vi "Random_Number.vi"() -> ()   [LabVIEW 2017]
panel:
  in  "stop":bool
  out "Waveform Chart":dbl(graph)
  out "Test Indicator":dbl
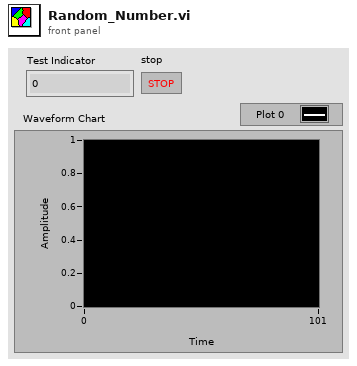
[diagram p1: front panel]
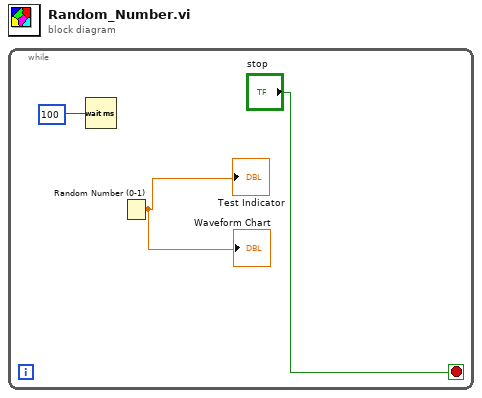
[diagram p0: block diagram]
diagram:
  n1 = while {
    stop <- "stop" stop-if-true
    n2 = Wait (ms)(milliseconds to wait=u32 100) -> ()  [unwired: 1 out]
    n3 = Random Number (0-1)() -> (number: 0 to 1=→"Test Indicator" →"Waveform Chart":dbl)
  }
